vi "AssertSubpanelVIExecCore.vi"(0 "VI Reference In":refnum<vi>, 1 "Label":string, 2 "delimiter (>>)":string=">>", 3 "Assert Only? (F)":bool, 5 "Control Path":string, 7 "Execution:State":T1(array[ring]), 11 "Error In":errorcluster, 12 "Assert Interval(10 ms)":u32=10, 13 "Timeout(5 sec)":dbl=5.0) -> (4 "VI Reference Out":refnum<vi>, 15 "Error Out":errorcluster)   [LabVIEW 2016, in "Drona.lvlib" / "AssertSubpanel.lvlib"]
doc: "Asserts the state of controls.\n\nThe input control name is given as a string , incase of path, use delimiters inbetween the path."
uses:
  AssertSubpanel.lvlib
  Get/GetControlRef/GetControlRefByPath.vi
  <vilib>/addons/_JKI Toolkits/Caraya/classes/Assert/Assert True.vi
  <vilib>/addons/_JKI Toolkits/Caraya/classes/Assert/Assert.lvclass
  Get/GetControlRef/GetControlRef.lvlib
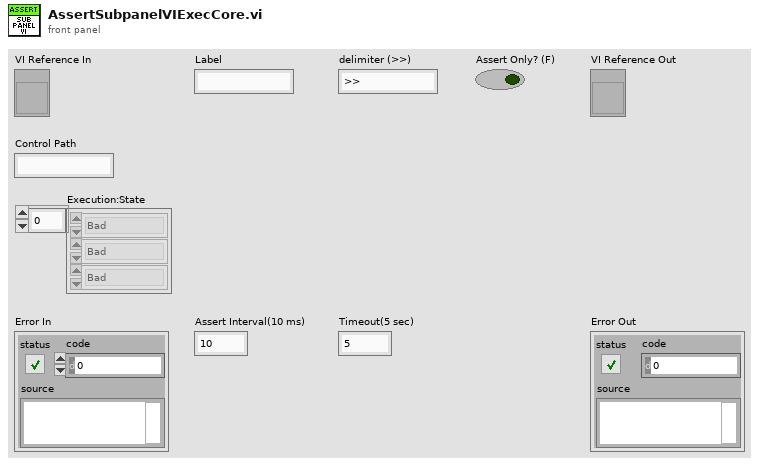
[diagram p1: front panel]
types:
  T1 = enum32{"Bad", "Idle", "Run top level", "Running"}[]
  T2 = enum32{"Bad", "Idle", "Run top level", "Running"}
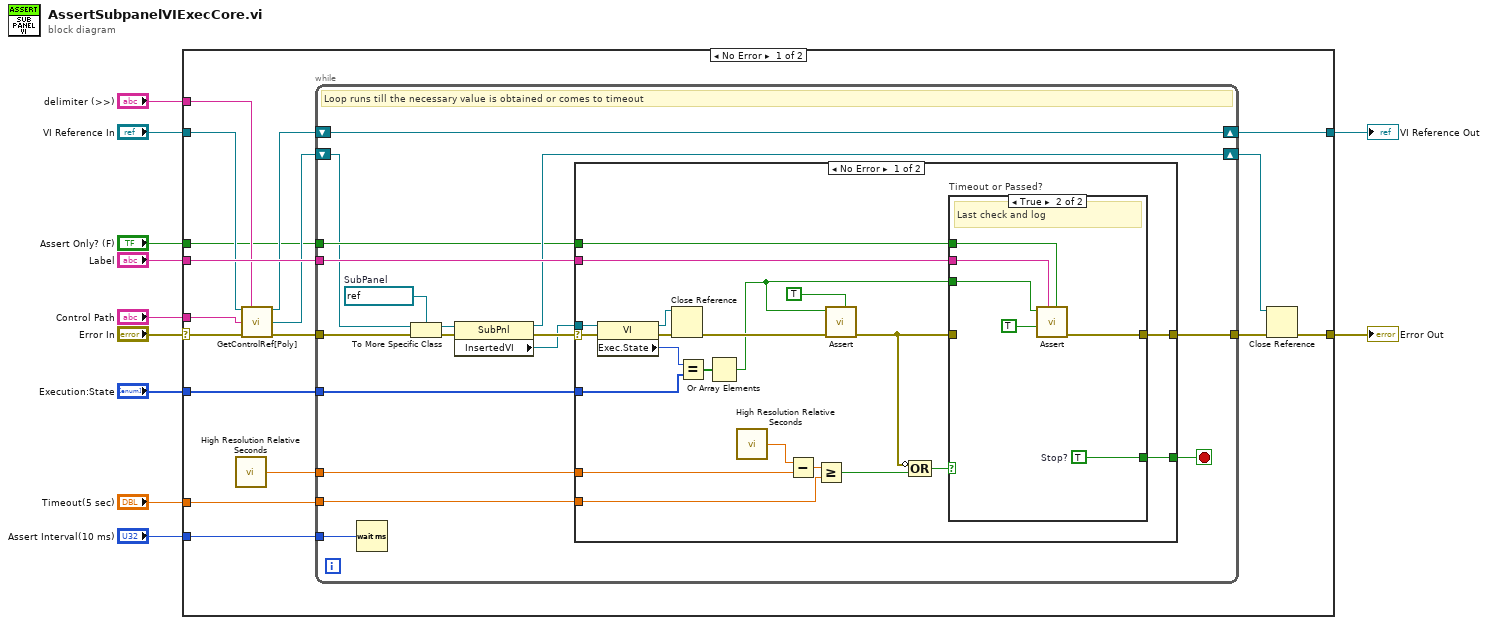
[diagram p0: block diagram]
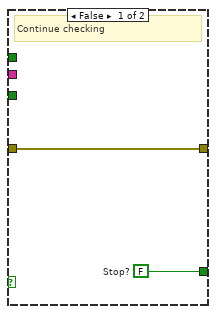
[diagram p2: hidden frame]
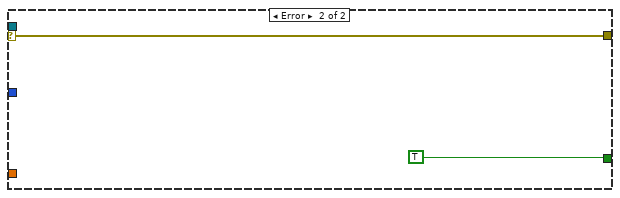
[diagram p3: hidden frame]
diagram:
  n1 = case shown="No Error" "Error In" {
    selector: "Error In" -> [w23 w78]
    tunnel: "Timeout(5 sec)" -> [w28 _]
    tunnel: [w27 w77] -> w10
    tunnel: [w16 w78] -> w9
    tunnel: "Assert Interval(10 ms)" -> [w25 _]
    tunnel: "Label" -> [w24 _]
    tunnel: "VI Reference In" -> [w22 w77]
    tunnel: "Control Path" -> [w21 _]
    tunnel: "delimiter (>>)" -> [w14 _]
    tunnel: "Assert Only? (F)" -> [w13 _]
    tunnel: "Execution:State" -> [w12 _]
    frame No Error {
      n2 = call <vilib>:"High Resolution Relative Seconds.vi"() -> ("relative seconds"=w20:dbl)
      n3 = call-poly "GetControlRef[Poly].vi"("VI Reference In"=w22, "delimiter (>>)"=w14, "Control Path"=w21, "error In"=w23) -> ("VI Reference Out"=w18:refnum<vi>, "Ctl Refnum"=w17:refnum<vi>, "error out"=w19:errorcluster)  [unwired: 9 in]
      n4 = while {
        tunnel: w28 -> [w44]
        tunnel: w20 -> [w45]
        tunnel: w19 -> [w39]
        tunnel: [w42] -> w26
        tunnel: w25 -> [w40]
        tunnel: w24 -> [w37]
        shift-right: [w38] -> w27
        shift-left: w18 -> [w38]
        shift-right: [w36] -> w15
        shift-left: w17 -> [w30]
        tunnel: w13 -> [w35]
        tunnel: w12 -> [w33]
        stop <- w43 stop-if-true
        w31 = refnum<vi> refnum  # SubPanel
        # "Loop runs till the necessary value is obtained or comes to timeout"
        n5 = Wait (ms)(milliseconds to wait=w40) -> ()  [unwired: 1 out]
        n6 = To More Specific Class(target class=w31, reference=w30, error in=w39) -> (specific class reference=w29:refnum<vi>, error out=w32:errorcluster)
        n7 = property class="SubPnl"(reference=w29, error in=w32) -> (reference out=w36:refnum<vi>, error out=w41:errorcluster, "InsertedVI"=w34:refnum<vi>)
        n8 = case shown="No Error" w41 {
          selector: w41 -> [w53 w76]
          tunnel: w45 -> [w66 _]
          tunnel: w44 -> [w63 _]
          tunnel: [w56 TRUE] -> w43
          tunnel: [w57 w76] -> w42
          tunnel: w34 -> [w54 _]
          tunnel: w37 -> [w62 _]
          tunnel: w35 -> [w55 _]
          tunnel: w33 -> [w48 _]
          frame No Error {
            n9 = property class="VI"(reference=w54, error in=w53) -> (reference out=w50:refnum<vi>, error out=w52:errorcluster, "Exec.State"=w49:T2)
            n10 = Close Reference(reference=w50, error in (no error)=w52) -> (error out=w51:errorcluster)
            n11 = Equal?(x=w49, y=w48) -> (x = y?=w47:bool[])
            n12 = Or Array Elements(Boolean array=w47) -> (logical OR=w46:bool)
            n13 = call <vilib>:"High Resolution Relative Seconds.vi"() -> ("relative seconds"=w65:dbl)
            n14 = Subtract(x=w65, y=w66) -> (x-y=w64:dbl)
            n15 = Greater Or Equal?(x=w64, y=w63) -> (x >= y?=w61:bool)
            n16 = call-poly <vilib>:"Assert.vi"("Assert Only? (F)"=TRUE, "error in (no error)"=w51, "True?"=w46) -> ("error out"=w60:errorcluster)  [unwired: 8 in]
            n17 = Compound Arithmetic op=OR(invert w60, w61) -> (w59:bool)
            n18 = case "Timeout or Passed?" shown="True" w59 {
              tunnel: w60 -> [w68 _]
              tunnel: w46 -> [_ w73]
              tunnel: w62 -> [_ w74]
              tunnel: [w68 w72] -> w57
              tunnel: [w67 w71] -> w56
              tunnel: w55 -> [_ w69]
              frame False {
                w67 = FALSE  # Stop?
                # "Continue checking"
              }
              frame True {
                w71 = TRUE  # Stop?
                # "Last check and log"
                n19 = call-poly <vilib>:"Assert.vi"("Assert Only? (F)"=w69, "Label"=w74, "Register with caller test (F)"=TRUE, "True?"=w73) -> ("error out"=w72:errorcluster)  [unwired: 7 in]
              }
            }
          }
          frame Error {
          }
        }
      }
      n20 = Close Reference(reference=w15, error in (no error)=w26) -> (error out=w16:errorcluster)
    }
    frame Error {
    }
  }
  "Error Out" <- w9
  "VI Reference Out" <- w10
